vi "generatore_sinusoide.vi"(0 "f0 (frequenza base) [Hz]":dbl min=0.0, 1 "Ap (ampiezza di picco)":dbl min=0.0, 2 "Tc (periodo di campionamento) [s]":dbl min=0.0, 3 "Ta (tempo di analisi) [s]":dbl min=0.0, 5 "Phi (fase iniziale) [rad]":dbl, 8 "DC Offset":dbl) -> (7 "Waveform Graph":waveform(dbl)(graph))   [LabVIEW 2009]
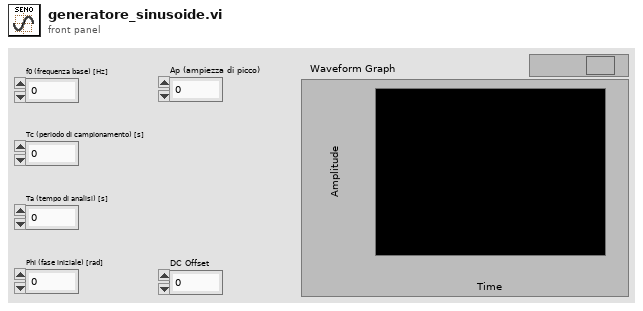
[diagram p1: front panel]
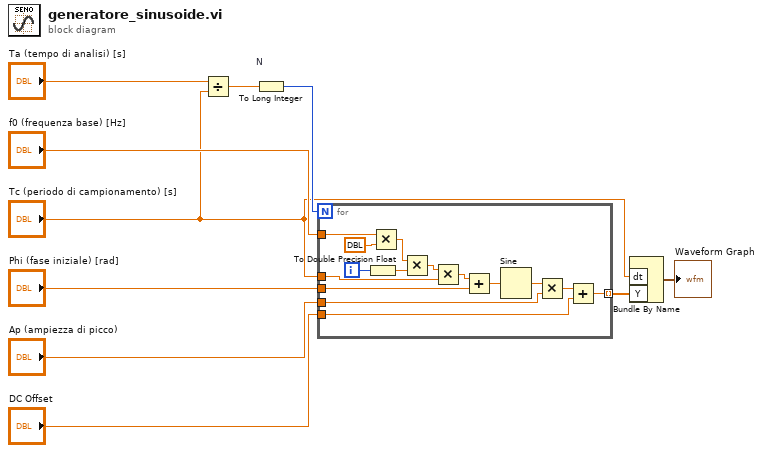
[diagram p0: block diagram]
diagram:
  n1 = Divide(x="Ta (tempo di analisi) [s]", y="Tc (periodo di campionamento) [s]") -> (x/y=w6:dbl)
  n2 = To Long Integer "N"(number=w6) -> (32bit integer=w7:i32)
  n3 = for {
    N: w7 -> [_]
    tunnel: "Phi (fase iniziale) [rad]" -> [w25]
    tunnel: "DC Offset" -> [w19]
    tunnel: "Ap (ampiezza di picco)" -> [w21]
    tunnel: "f0 (frequenza base) [Hz]" -> [w24]
    tunnel: "Tc (periodo di campionamento) [s]" -> [w23]
    tunnel: [w18] -> w4 mode=indexing
    i -> [w17]
    n4 = To Double Precision Float(number=w17) -> (double precision float=w14:dbl)
    n5 = Multiply(x=w24, y=dbl ?) -> (x*y=w15:dbl)
    n6 = Multiply(x=w15, y=w14) -> (x*y=w13:dbl)
    n7 = Multiply(x=w13, y=w23) -> (x*y=w12:dbl)
    n8 = Add(x=w12, y=w25) -> (x+y=w11:dbl)
    n9 = Sine(x=w11) -> (sin(x)=w22:dbl)
    n10 = Multiply(x=w22, y=w21) -> (x*y=w20:dbl)
    n11 = Add(x=w20, y=w19) -> (x+y=w18:dbl)
  }
  n12 = Bundle By Name("dt"="Tc (periodo di campionamento) [s]", "Y"=w4) -> (→"Waveform Graph":waveform(dbl))  [unwired: 1 in]
